vi "ChooseCam.vi"() -> (3 "Array of Cams":string[](array[string]), 4 "Cam":string, 5 "PicoPad":string, 6 "Config File 2":path)   [LabVIEW 2013]
panel:
  in  "Config File":path
  in  "choose Pico":u16(ring) items=["PicoPad3", "PicoPad4"]
  in  "stop":bool
  in  "choose cam":u16(ring) items=["10TW_Driver_Spot_Cam", "B1_TelInput", "B2_TelLens1", "B5_CompressorOut", "B6_SwitchYNear", "GIGEtest", "L3_TelescopeOut", "L4_TREXpass1", "L5_TREXPass2", "L6_TREXpass3", "L7_TREXPass4", "L8_M10Leak", "OAPtestCam", "PaperCam", "StagingAlignBeam1", "StagingAlignBeam2", "StagingCapAlignment", "StagingCapSpec", "StagingCapSpec1stOrder", "StagingChromaxGuppy", "StagingDiodeMonitor", "StagingFocusBeam1", "StagingFocusBeam2", "StagingGuppy", "StagingM1Far", "StagingM1Near", "StagingM3Far", "StagingM4", "StagingM5", "StagingMagnetCam1", "StagingMagnetCam2", "StagingMagnetCam3", "StagingManta2", "StagingModeImager2", "StagingModeTemp", "StagingOAP1Far", "StagingOAP1Near", "StagingOAP2Far", "StagingOAP2Near", "StagingPhasics", "StagingPhosphor", "StagingTapeCam", "StagingTapeMonitorCam", "TargetCam10Hz_Diode", "TREXVarianCam0", "TREXVarianCam1", "TREXVarianCam2", "TREXVarianCam3", "TREX_CapSideView", "TREX_TA6", "TS-253a_in", "TS-CapSideview", "TS-CapSpec", "TS-ChromexCam", "TS-InputNearField", "TS-Mode1", "TS-OverlapCam", "TS-Periscope", "XUV_Cam1", "XUV_Cam2"]
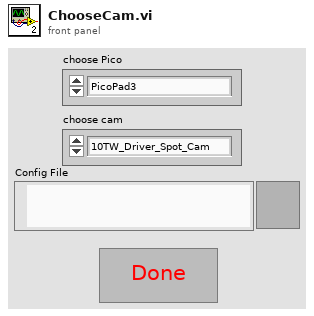
[diagram p1: front panel]
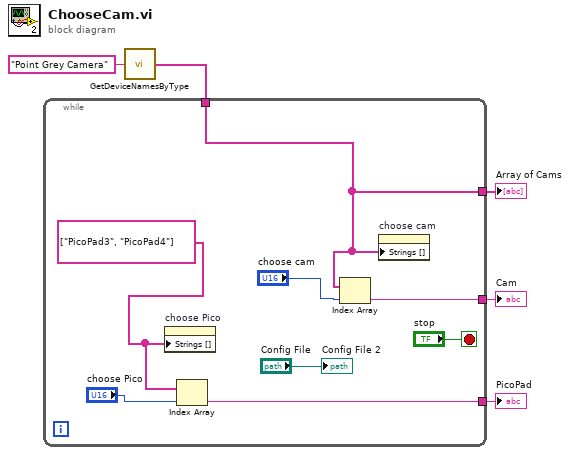
[diagram p0: block diagram]
diagram:
  n1 = call "GetDeviceNamesByType.vi"("Device Type"="Point Grey Camera") -> ("Array"=w1:string[])
  n2 = while {
    tunnel: [w12] -> w5
    tunnel: [w6] -> w4
    tunnel: [w8] -> w3
    tunnel: w1 -> [w6]
    stop <- "stop" stop-if-true
    w10 = string[] ["PicoPad3", "PicoPad4"] ("Array")
    n3 = property on="choose Pico" class="Ring (strict)"("Strings []"=w10) -> ()  [unwired: 2 in, 2 out]
    n4 = Index Array(array=w10, index="choose Pico") -> (element=w8:string)
    n5 = Index Array(array=w6, index="choose cam") -> (element=w12:string)
    n6 = property on="choose cam" class="Ring (strict)"("Strings []"=w6) -> ()  [unwired: 2 in, 2 out]
    "Config File 2" <- "Config File"
  }
  "Cam" <- w5
  "Array of Cams" <- w4
  "PicoPad" <- w3
